vi "Open.vi"(8 "error in (no error)":errorcluster, 10 "name (unnamed)":string, 11 "Message Queue in":refnum<class "Message Queue.lvclass">) -> (0 "error out":errorcluster, 3 "Message Queue out":refnum<class "Message Queue.lvclass">)   [LabVIEW 2027, in "Messaging.lvlib" / "Message Queue.lvclass"]
uses:
  Message Queue.lvclass
  Message Queue.lvclass/Message Queue.ctl
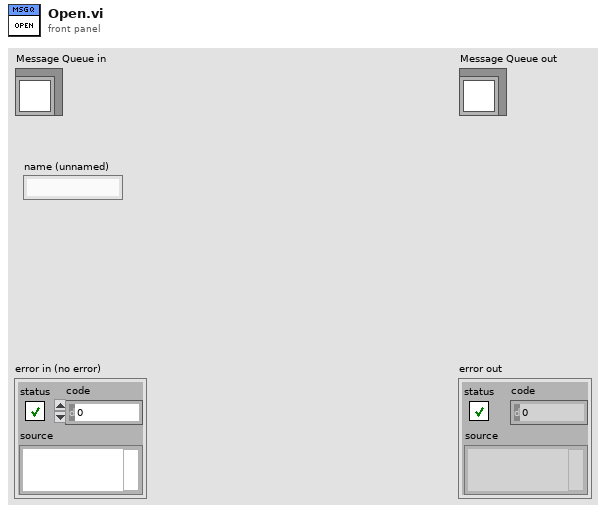
[diagram p1: front panel]
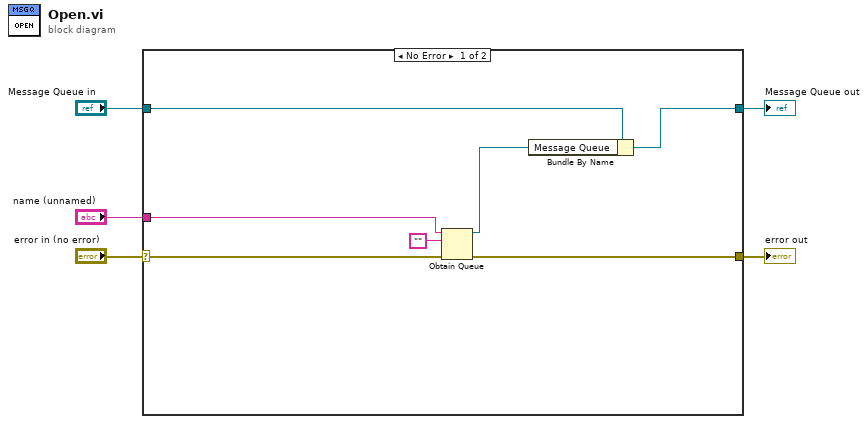
[diagram p0: block diagram]
diagram:
  n1 = case shown="No Error" "error in (no error)" {
    selector: "error in (no error)" -> [w12 w14]
    tunnel: [w11 w14] -> w4
    tunnel: [w8 w13] -> w2
    tunnel: "Message Queue in" -> [w9 w13]
    tunnel: "name (unnamed)" -> [w10 _]
    frame No Error {
      n2 = Obtain Queue(name (unnamed)=w10, element data type="", error in (no error)=w12) -> (queue out=w6:refnum<queue>, error out=w11:errorcluster)  [unwired: 2 in, 1 out]
      n3 = Bundle By Name(cluster=w9, "Message Queue"=w6) -> (w8:refnum<class "Message Queue.lvclass">)
    }
    frame Error {
    }
  }
  "error out" <- w4
  "Message Queue out" <- w2
